vi "SMU_Only4Wire Resistance.vi"(6 "current level":dbl=0.01 format="%_6p", 8 "error in (no error)":errorcluster, 9 "Published Data Id":string, 10 "Pins":string[](array[string]), 11 "Semiconductor Module Context":T1) -> (0 "error Out":errorcluster, 2 "R Array":dbl[](array[numeric]), 3 "Semiconductor Module Context Out":T1)   [LabVIEW 2013]
uses:
  <vilib>/NI_TestStand_SemiconductorModule/NI_TestStand_Semiconductor_Module.lvlibp/PinMap/General/SemiconductorModuleContext.ctl
  <vilib>/NI_TestStand_SemiconductorModule/NI_TestStand_Semiconductor_Module.lvlibp/PinMap/DC Power/PinsToNIDCPowerSessions.vi
  <vilib>/NI_TestStand_SemiconductorModule/NI_TestStand_Semiconductor_Module.lvlibp/PinMap/General/Publish/PublishDataDoubleFunctionalTest.vi
  <vilib>/NI_TestStand_SemiconductorModule/NI_TestStand_Semiconductor_Module.lvlibp
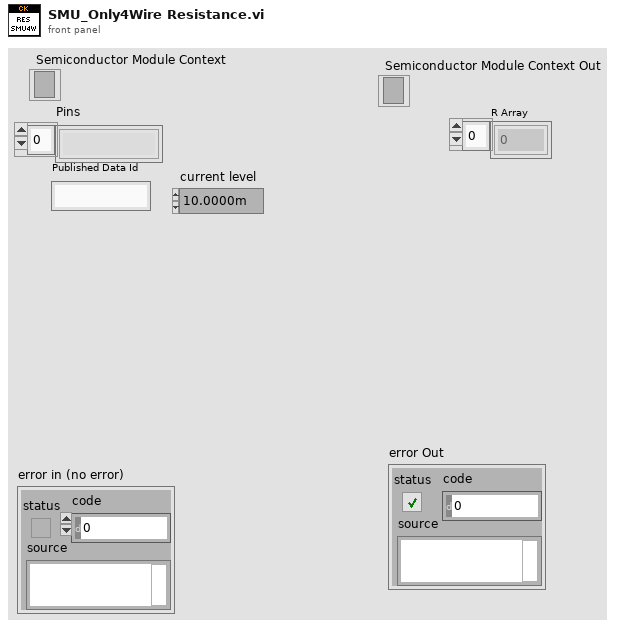
[diagram p1: front panel]
types:
  T1 = typedef "NI_TestStand_Semiconductor_Module.lvlibp/SemiconductorModuleContext.ctl" = refnum<k7>
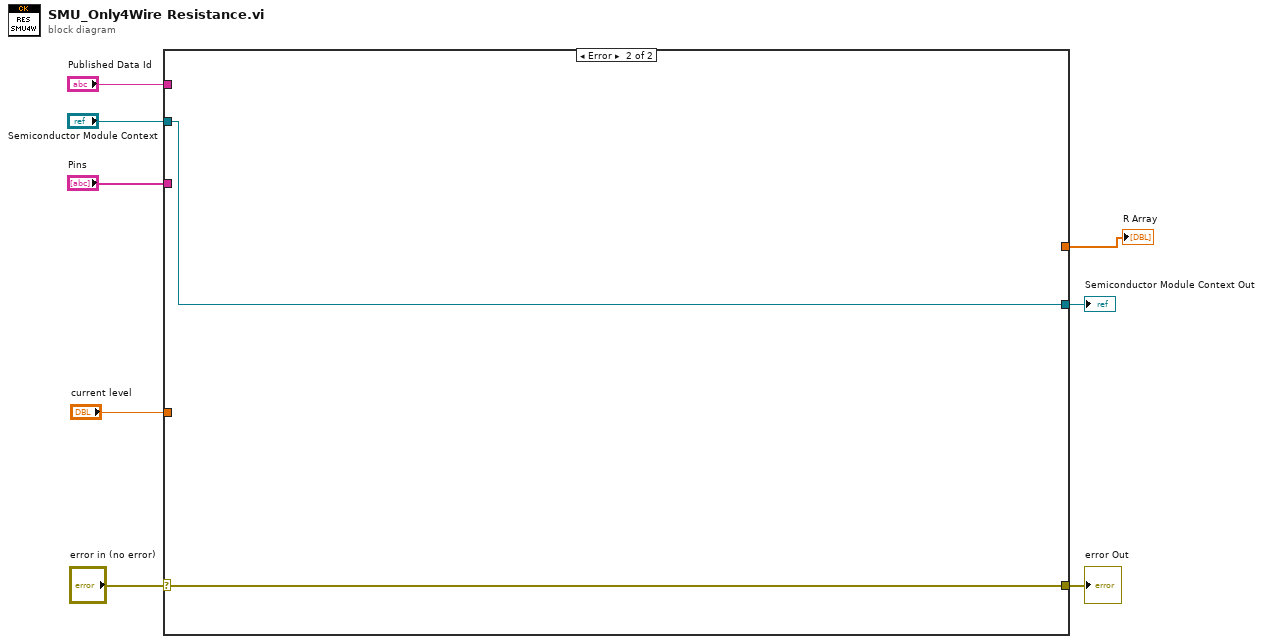
[diagram p0: block diagram]
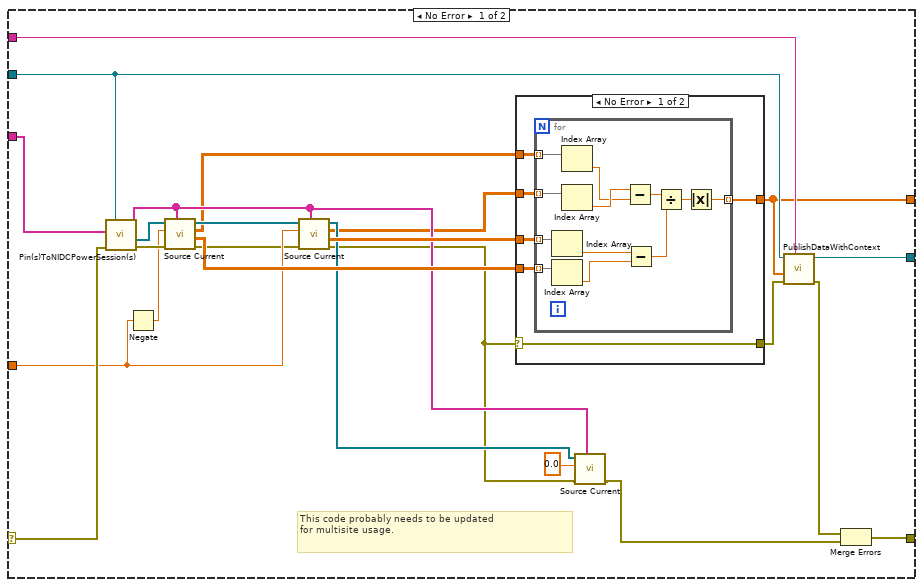
[diagram p2: hidden frame]
diagram:
  n1 = case shown="Error" "error in (no error)" {
    selector: "error in (no error)" -> [w31 w53]
    tunnel: "Semiconductor Module Context" -> [w13 w52]
    tunnel: "Pins" -> [w17 _]
    tunnel: [w28 w53] -> w5
    tunnel: "Published Data Id" -> [w32 _]
    tunnel: "current level" -> [w20 _]
    tunnel: [w18 w52] -> w2
    tunnel: [w9 _] -> w1
    frame No Error {
      # "This code probably needs to be updated\nfor multisite usage."
      n2 = call-poly <vilib>:"Pin(s)ToNIDCPowerSession(s).vi"("error in (no error)"=w31, "Pins"=w17, "Semiconductor Module Context"=w13) -> ("error out"=w24:errorcluster, "Instrument Sessions"=w25:refnum<k15>[], "Channel Lists"=w16:string[])  [unwired: 4 in, 2 out]
      n3 = Negate(x=w20) -> (-x=w19:dbl)
      n4 = call "Source Current.vi"("Channel Lists"=w16, "error in (no error)"=w24, "current level"=w19, "Instrument Sessions In"=w25) -> ("error out"=w12:errorcluster, "current measurements"=w26:dbl[][], "voltage measurements"=w10:dbl[][], "Instrument Sessions Out"=w11:refnum<k15>[])  [unwired: 4 in]
      n5 = call "Source Current.vi"("Channel Lists"=w16, "error in (no error)"=w12, "current level"=w20, "Instrument Sessions In"=w11) -> ("error out"=w15:errorcluster, "current measurements"=w27:dbl[][], "voltage measurements"=w14:dbl[][], "Instrument Sessions Out"=w22:refnum<k15>[])  [unwired: 4 in]
      n6 = case shown="No Error" w15 {
        selector: w15 -> [w35 w51]
        tunnel: w14 -> [w38 _]
        tunnel: w27 -> [w37 _]
        tunnel: [w36 _] -> w9
        tunnel: [w35 w51] -> w30
        tunnel: w26 -> [w34 _]
        tunnel: w10 -> [w33 _]
        frame No Error {
          n7 = for {
            tunnel: w38 -> [w42] mode=indexing
            tunnel: w37 -> [w50] mode=indexing
            tunnel: [w48] -> w36 mode=indexing
            tunnel: w34 -> [w46] mode=indexing
            tunnel: w33 -> [w39] mode=indexing
            n8 = Index Array(array=w50) -> (element=w43:dbl)  [unwired: 1 in]
            n9 = Index Array(array=w46) -> (element=w45:dbl)  [unwired: 1 in]
            n10 = Index Array(array=w39) -> (element=w40:dbl)  [unwired: 1 in]
            n11 = Index Array(array=w42) -> (element=w41:dbl)  [unwired: 1 in]
            n12 = Subtract(x=w41, y=w40) -> (x-y=w47:dbl)
            n13 = Subtract(x=w43, y=w45) -> (x-y=w44:dbl)
            n14 = Divide(x=w47, y=w44) -> (x/y=w49:dbl)
            n15 = Absolute Value(x=w49) -> (abs(x)=w48:dbl)
          }
        }
        frame Error {
        }
      }
      n16 = call "Source Current.vi"("Channel Lists"=w16, "error in (no error)"=w15, "current level"=0.0, "Instrument Sessions In"=w22) -> ("error out"=w23:errorcluster)  [unwired: 4 in, 3 out]
      n17 = call-poly <vilib>:"PublishDataWithContext.vi"("Published Data Id"=w32, "error in (no error)"=w30, "Data In"=w9, "Semiconductor Module Context"=w13) -> ("error out"=w29:errorcluster, "Semiconductor Module Context Out"=w18:T1)  [unwired: 6 in]
      n18 = Merge Errors(w29, w23) -> (w28:errorcluster)
    }
    frame Error {
    }
  }
  "error Out" <- w5
  "Semiconductor Module Context Out" <- w2
  "R Array" <- w1
